vi "Test_Config.vi"() -> ()   [LabVIEW 2016]
uses:
  Libraries/OBJ-Serial/Controls/Cmd_Rx.ctl
  Libraries/OBJ-Serial/Controls/PortConfig.ctl
  Libraries/OBJ-Serial/Serial_G.lvlib
  Libraries/OBJ-GPS/NMEA.lvlib
panel:
  in  "Stop":bool
  in  "Rx":bool
  out "Read":T1
  out "CheckSumOk?":bool
  out "GPRMC":string
  out "GPGSV":string
  out "GPGSA":string
  out "GPGGA":string
  out "GPVTG":string
  out "Resp":string
  out "Port?":bool
  in  "error in":errorcluster
  in  "Port":string="COM13"
  out "error out":errorcluster
  # "Serial Rx"
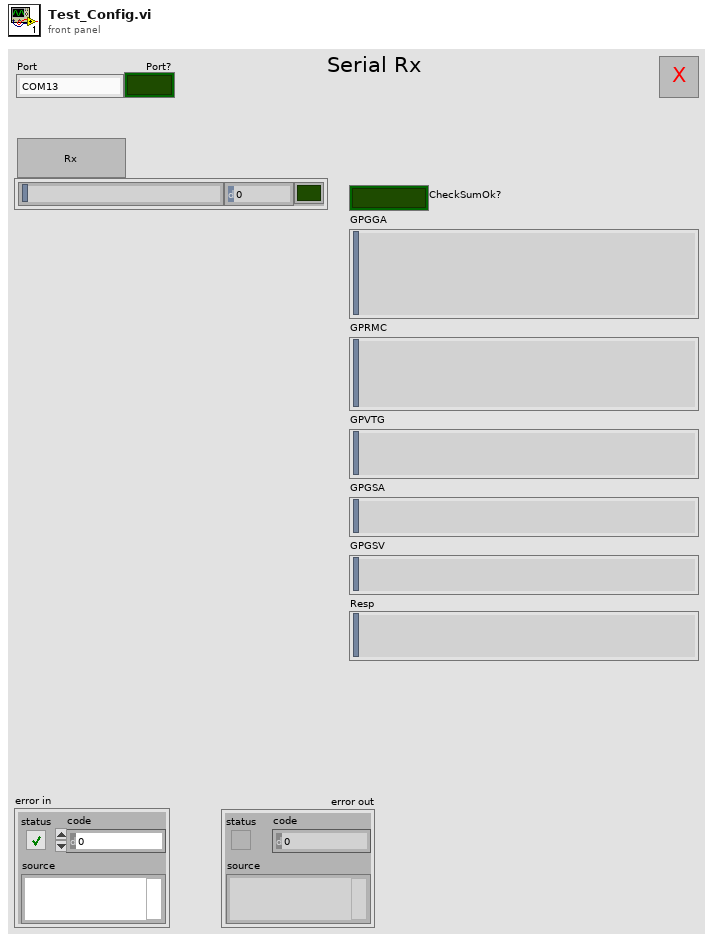
[diagram p1: front panel]
types:
  T1 = typedef "Serial_G.lvlib/Cmd_Rx.ctl" = cluster{"Read":string, "ExecTime (ms)":i32, "Timeout?":bool}
  T2 = typedef "Serial_G.lvlib/PortConfig.ctl" = cluster{"Baud rate":u32, "Parity":enum16{"None", "Odd", "Even", "Mark", "Space"}, "Data bits":u16, "Stop bits":u16, "Flow control":u16}
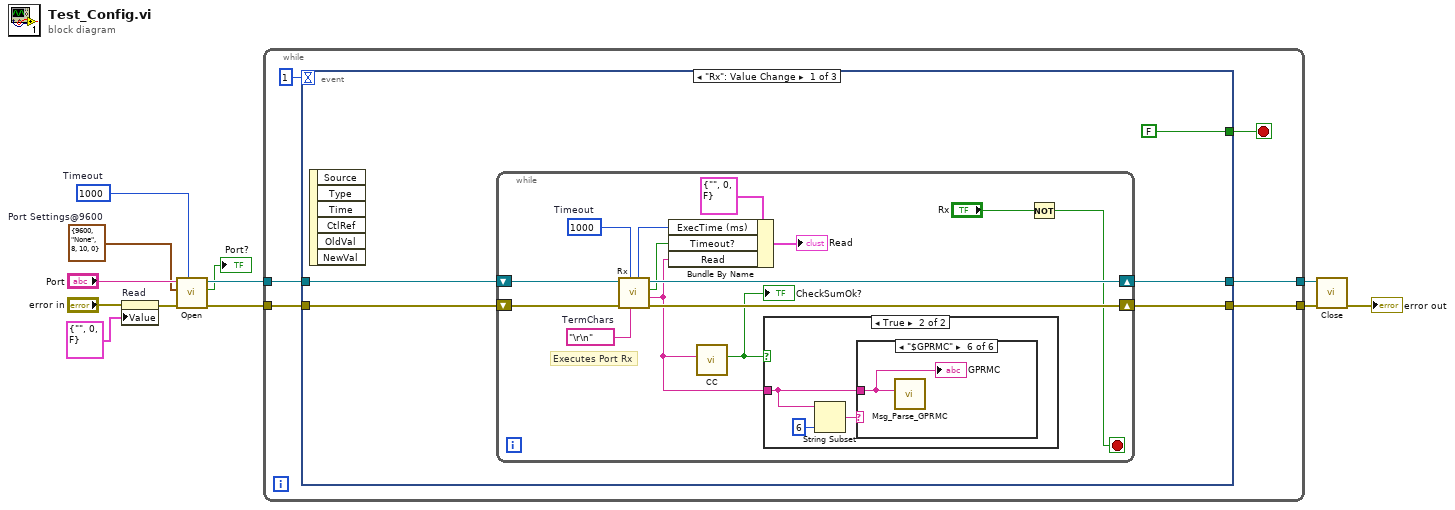
[diagram p0: block diagram]
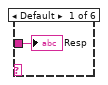
[diagram p3: hidden frame]
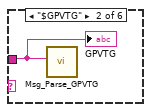
[diagram p4: hidden frame]
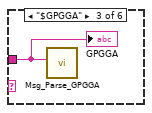
[diagram p5: hidden frame]
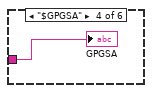
[diagram p6: hidden frame]
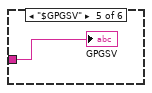
[diagram p7: hidden frame]
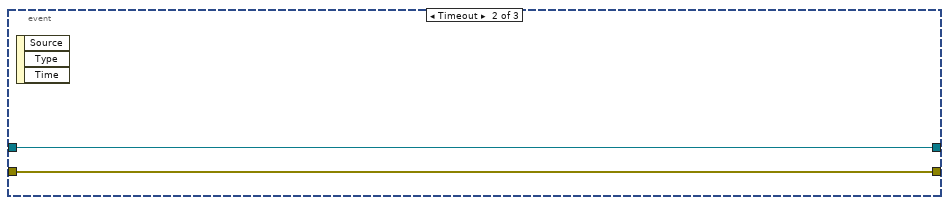
[diagram p8: hidden frame]
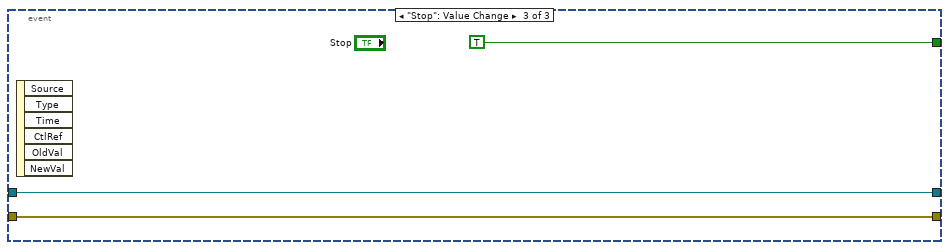
[diagram p9: hidden frame]
diagram:
  w1 = u32 1000  # Timeout
  w2 = T2 {"Baud rate"=9600, "Parity"=enum."None", "Data bits"=8, "Stop bits"=10, "Flow control"=0}  # Port Settings@9600
  n1 = property on="Read" class="Clust (strict)"(error in="error in", "Value"=T1 {"Read"="", "ExecTime (ms)"=0, "Timeout?"=FALSE} ("Read")) -> (error out=w5:errorcluster)  [unwired: 1 in, 1 out]
  n2 = call "Open.vi"("Timeout (3000)"=w1, "error in"=w5, "ConfigPort (9600,0,8,1)"=w2, "Port(Alias)"="Port") -> ("error out"=w12:errorcluster, "PortFound?"=→"Port?":bool, "VISA out"=w11:refnum<visa-resource-name>)  [unwired: 4 in, 1 out]
  n3 = while {
    tunnel: w11 -> [w17]
    tunnel: [w16] -> w10
    tunnel: w12 -> [w18]
    tunnel: [w15] -> w8
    stop <- w14 stop-if-true
    n4 = event shown="[0] \"Rx\": Value Change" {
      selector: _ -> [_ _ _]
      dyn-events: _ -> [_ _ _]
      timeout: 1 -> [_ _ _]
      tunnel: w18 -> [w23 w47 w50]
      tunnel: w17 -> [w22 w48 w49]
      tunnel: [w21 w48 w49] -> w16
      tunnel: [w20 w47 w50] -> w15
      tunnel: [FALSE ("Rx") _ TRUE ("Rx")] -> w14
      event "Rx": Value Change {
        n5 = event-data() -> ()  [unwired: 1 in, 6 out]
        n6 = while {
          shift-right: [w34] -> w20
          shift-left: w23 -> [w37]
          shift-right: [w35] -> w21
          shift-left: w22 -> [w36]
          stop <- w24 stop-if-true
          w26 = u32 1000  # Timeout
          w30 = "\r\n"  # TermChars
          # "Executes Port Rx"
          n7 = call "Rx.vi"("Wait for? (\\r\\n)"=w30, "Timeout_ms (3000)"=w26, "error in"=w37, "VISA in"=w36) -> ("error out"=w34:errorcluster, "Response"=w28:string, "Timeout?"=w32:bool, "VISA out"=w35:refnum<visa-resource-name>, "ExecTime(ms)"=w31:i32)  [unwired: 3 in]
          n8 = Bundle By Name(cluster=T1 {"Read"="", "ExecTime (ms)"=0, "Timeout?"=FALSE} ("Read"), "ExecTime (ms)"=w31, "Timeout?"=w32, "Read"=w28) -> (→"Read":T1)
          n9 = call "CC.vi"("Sentence"=w28) -> ("CheckSumOk?"=w27:bool)  [unwired: 9 in, 1 out]
          "CheckSumOk?" <- w27
          n10 = case shown="True" w27 {
            tunnel: w28 -> [_ w38]
            frame False {
            }
            frame True {
              n11 = String Subset(string=w38, length (rest)=6 ("length (rest)")) -> (substring=w39:string)  [unwired: 1 in]
              n12 = case shown="\"$GPRMC\"" w39 {
                tunnel: w38 -> [w41 w42 w43 w44 w45 w46]
                frame Default {
                  "Resp" <- w41
                }
                frame "$GPVTG" {
                  n13 = call "Msg_Parse_GPVTG.vi"("$GPVTG-message_IN"=w42) -> ()  [unwired: 9 in, 2 out]
                  "GPVTG" <- w42
                }
                frame "$GPGGA" {
                  n14 = call "Msg_Parse_GPGGA.vi"("$GPGGA-message_IN"=w43) -> ()  [unwired: 9 in, 2 out]
                  "GPGGA" <- w43
                }
                frame "$GPGSA" {
                  "GPGSA" <- w44
                }
                frame "$GPGSV" {
                  "GPGSV" <- w45
                }
                frame "$GPRMC" {
                  n15 = call "Msg_Parse_GPRMC.vi"("$GPRMC-message_IN"=w46) -> ()  [unwired: 9 in, 2 out]
                  "GPRMC" <- w46
                }
              }
            }
          }
          n16 = Not(x="Rx") -> (.not. x?=w24:bool)
        }
      }
      event Timeout {
        n17 = event-data() -> ()  [unwired: 1 in, 3 out]
      }
      event "Stop": Value Change {
        n18 = event-data() -> ()  [unwired: 1 in, 6 out]
      }
    }
  }
  n19 = call "Close.vi"("error in"=w8, "VISA in"=w10) -> ("error out"=→"error out":errorcluster)  [unwired: 9 in]
